vi "Panel Create.vi"(10 "Panel":refnum<class "Helper Loop.lvclass">, 11 "Dev Actor in":refnum<class "Dev Actor.lvclass">) -> (3 "Dev Actor out":refnum<class "Dev Actor.lvclass">)   [LabVIEW 2021, in "Dev Actor.lvlib" / "Dev Actor.lvclass"]
uses:
  Dev Actor.lvclass
  Helper Loop/Helper Loop.lvclass
  Dev Actor.lvclass/Dev Actor.ctl
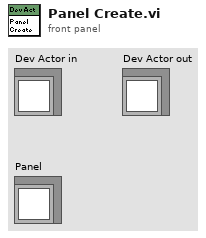
[diagram p1: front panel]
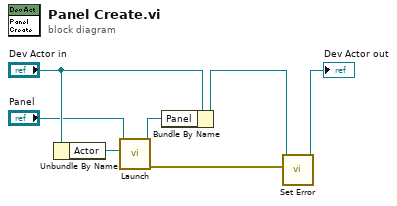
[diagram p0: block diagram]
diagram:
  n1 = Unbundle By Name("Dev Actor in") -> ("Actor"=w2:refnum<class "Actor.lvclass">)
  n2 = call "Launch.vi"("Actor"=w2, "Panel in"="Panel") -> ("error out"=w6:errorcluster, "Panel out"=w7:refnum<class "Helper Loop.lvclass">)  [unwired: 8 in]
  n3 = Bundle By Name(cluster="Dev Actor in", "Panel"=w7) -> (w5:refnum<class "Dev Actor.lvclass">)
  n4 = call-dynamic "Set Error.vi"("Merge"=w6, "Dev Actor in"=w5) -> ("Dev Actor out"=→"Dev Actor out":refnum<class "Dev Actor.lvclass">)  [unwired: 9 in]
